vi "PH_gentec_M-Link.Action get Info.vi"(0 "i ref in":refnum<vi>, 5 "error in":errorcluster) -> (14 "i ref out":refnum<vi>, 19 "error out":errorcluster)   [LabVIEW 2014, in "PH_gentec_M-Link.lvlib"]
doc: "This VI gets the basic information from the device."
uses:
  PH_gentec_M-Link.lvlib
  non_GPL/instr.lib/gentec-M-LINK/Driver/Type Defs/gentec-M-Link.Sensor Type.ctl
  non_GPL/instr.lib/gentec-M-LINK/Driver/Type Defs/gentec-M-Link.Range.ctl
  non_GPL/instr.lib/gentec-M-LINK/Driver/Type Defs/gentec-M-Link.Queries with String Answers.ctl
  non_GPL/instr.lib/gentec-M-LINK/Driver/Type Defs/gentec-M-Link.Range Queries.ctl
  PH_Powermeter_BaseClass/PH_Powermeter_BaseClass.State.ctl
  PH_Powermeter_BaseClass/PH_Powermeter_BaseClass.Head Attributes.ctl
  non_GPL/instr.lib/gentec-M-LINK/gentec-M-Link - Driver.lvlib
  PH_Powermeter_BaseClass/PH_Powermeter_BaseClass.lvlib
panel:
  in  "Dummy":T1 items=["1f", "3f", "10f", "30f", "100f", "300f", "1p", "3p", "10p", "30p", "100p", "300p", "1n", "3n", "10n", "30n", "100n", "300n", "1u", "3u", "10u", "30u", "100u", "300u", "1m", "3m", "10m", "30m", "100m", "300m", "1", "3", "10", "30", "100", "300", "1K", "3K", "10K", "30K", "100K", "300K", "1M", "3M", "10M", "30M", "100M", "300M"]
  in  "Sensor Type":T2=1 items=["unknown", "Radiometer", "Joule Meter", "Optical Power", "Thermopyle Power"]
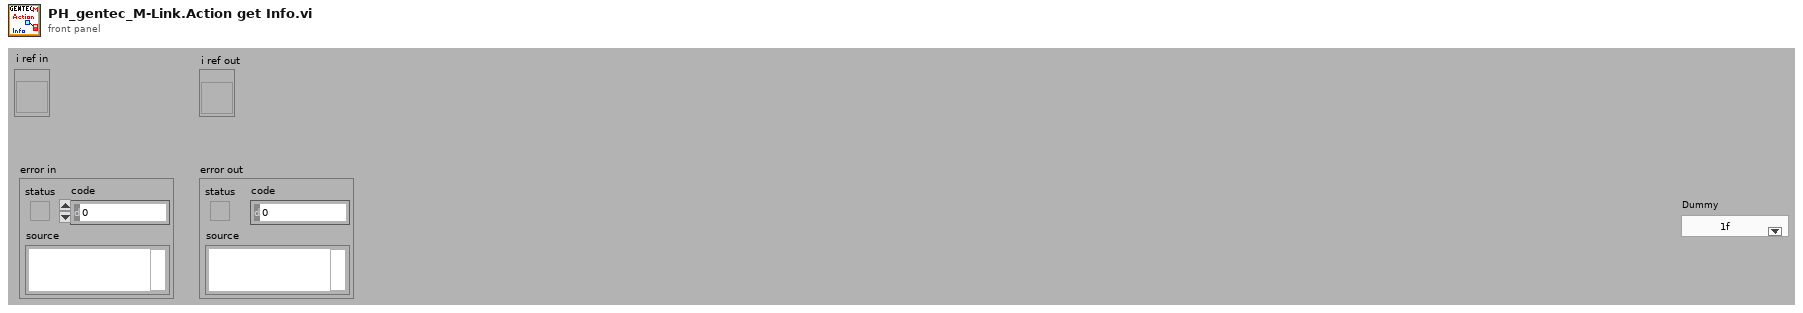
[diagram p1: front panel]
types:
  T1 = typedef "gentec-M-Link - Driver.lvlib/gentec-M-Link.Range.ctl" = u16
  T2 = typedef "gentec-M-Link - Driver.lvlib/gentec-M-Link.Sensor Type.ctl" = u16
  T3 = typedef "PH_Powermeter_BaseClass.lvlib/PH_Powermeter_BaseClass.Head Attributes.ctl" = cluster{"Instrument Type":string, "Head Version":string, "Head Name":string, "Serial Number":string, "Firmware":string, "Sensor Type":string, "MinimumRange":u32, "Maximum Range":u32, "Min Wavelength":i32, "Max Wavelength":i32}
  T4 = typedef "PH_Powermeter_BaseClass.lvlib/PH_Powermeter_BaseClass.State.ctl" = enum32{"off", "operating", "opened", "checked", "connected", "Sets to change", "running"}
  T5 = typedef "gentec-M-Link - Driver.lvlib/gentec-M-Link.Range Queries.ctl" = string
  T6 = typedef "gentec-M-Link - Driver.lvlib/gentec-M-Link.Queries with String Answers.ctl" = string
  T7 = typedef "PH_Powermeter_BaseClass.lvlib/PH_Powermeter_BaseClass.i attribute.ctl" = cluster{"GUI References":T8, "Connection":T9, "Head Attributes":T3, "VISA resource":refnum<visa-resource-name>, "Energy":T10, "Service ID Energy":i32, "Wanted Settings":T11, "Current Settings":T11}
  T8 = typedef "PH_Powermeter_BaseClass.lvlib/PH_Powermeter_BaseClass.GUI Refs.ctl" = cluster{"Head Attributes":refnum<vi>, "Energy":refnum<vi>, "Connection":refnum<vi>, "VISA Resource":refnum<vi>, "Energy evolution":refnum<vi>, "Scaling Factor":refnum<vi>, "Range":refnum<vi>, "Wavelength":refnum<vi>, "Trigger Level":refnum<vi>, "Wanted Settings":refnum<vi>, "Current Settings":refnum<vi>}
  T9 = typedef "PH_Powermeter_BaseClass.lvlib/PH_Powermeter_BaseClass.Connection.ctl" = cluster{"failed checks":i8, "Timeout":bool, "Data read":string, "Failure":bool, "Error":bool, "State":T4}
  T10 = typedef "PH_Powermeter_BaseClass.lvlib/PH_Powermeter_BaseClass.Energy.ctl" = cluster{"current Value":dbl, "unscaled":dbl, "Scaling Factor":dbl}
  T11 = typedef "PH_Powermeter_BaseClass.lvlib/PH_gentec_BaseClass.Head Settings.ctl" = cluster{"Trigger Level":dbl, "Wavelength":u32, "Range":u32}
  T12 = typedef "LVStringsAndValuesArrayTypeDef_U16.ctl" = cluster{"String":string, "Value":u16}[]
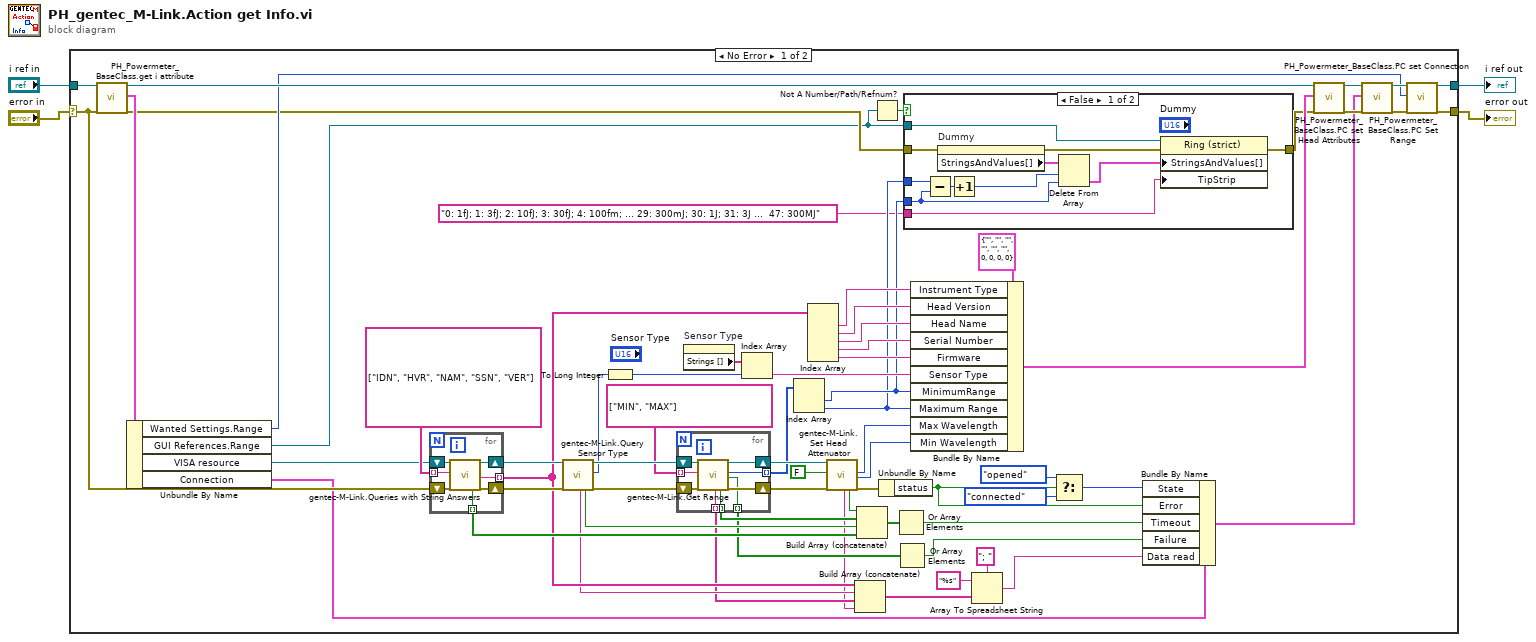
[diagram p0: block diagram]
diagram:
  n1 = case shown="No Error" "error in" {
    selector: "error in" -> [w26 w99]
    tunnel: [w15 w99] -> w3
    tunnel: "i ref in" -> [w27 w98]
    tunnel: [w13 w98] -> w1
    frame No Error {
      n2 = call "PH_Powermeter_BaseClass.get i attribute.vi"("i ref in"=w27, "error in (no error)"=w26) -> ("i ref out"=w25:refnum<vi>, "i attribute"=w20:T7, "error out"=w11:errorcluster)  [unwired: 15 in]
      n3 = Unbundle By Name(w20) -> ("Wanted Settings.Range"=w12:u32, "GUI References.Range"=w6:refnum<vi>, "VISA resource"=w19:refnum<visa-resource-name>, "Connection"=w18:T9)
      n4 = for {
        shift-right: [w97] -> w69
        shift-left: w26 -> [w96]
        shift-right: [w94] -> w68
        shift-left: w19 -> [w95]
        tunnel: [w93] -> w61 mode=indexing
        tunnel: T6[] ["IDN", "HVR", "NAM", "SSN", "VER"] -> [w92] mode=indexing
        tunnel: [w91] -> w43 mode=indexing
        n5 = call "gentec-M-Link.Queries with String Answers.vi"("VISA resource In"=w95, "Queries with String Answers"=w92, "error in (no error)"=w96) -> ("Read Timeout"=w93:bool, "VISA resource Out"=w94:refnum<visa-resource-name>, "Answer"=w91:string, "error out"=w97:errorcluster)  [unwired: 13 in]
      }
      n6 = call "gentec-M-Link.Query Sensor Type.vi"("VISA resource In"=w68, "error in (no error)"=w69) -> ("Data Read"=w42:string, "Read Timeout"=w60:bool, "VISA resource Out"=w67:refnum<visa-resource-name>, "Sensor Type"=w34:T2, "error out"=w65:errorcluster)  [unwired: 13 in]
      n7 = To Long Integer(number=w34) -> (32bit integer=w32:i32)
      n8 = for {
        shift-right: [w89] -> w66
        shift-left: w67 -> [w90]
        shift-right: [w87] -> w64
        shift-left: w65 -> [w88]
        tunnel: [w86] -> w59 mode=indexing
        tunnel: T5[] ["MIN", "MAX"] -> [w85] mode=indexing
        tunnel: [w84] -> w46 mode=indexing
        tunnel: [w83] -> w45 mode=indexing
        tunnel: [w82] -> w41 mode=indexing
        n9 = call "gentec-M-Link.Get Range.vi"("VISA resource In"=w90, "Range Queries"=w85, "error in (no error)"=w88) -> ("Data Read"=w82:string, "Read Timeout"=w86:bool, "VISA resource Out"=w89:refnum<visa-resource-name>, "Range"=w84:T1, "Error"=w83:bool, "error out"=w87:errorcluster)  [unwired: 11 in]
      }
      n10 = property on="Sensor Type" class="Ring (strict)"() -> ("Strings []"=w35:string[])  [unwired: 2 in, 2 out]
      n11 = Index Array(array=w35, index=w32) -> (element=w33:string)
      n12 = Index Array(array=w46) -> (element #1=w9:T1, element #2=w8:T1)  [unwired: 2 in]
      n13 = Index Array(array=w43) -> (element #1=w53:string, element #2=w52:string, element #3=w51:string, element #4=w50:string, element #5=w49:string)  [unwired: 5 in]
      n14 = call "gentec-M-Link.Set Head Attenuator.vi"("VISA resource In"=w66, "Set Head Attenuator"=FALSE, "error in (no error)"=w64) -> ("Data Read"=w40:string, "Read Timeout"=w58:bool, "Max Lambda"=w47:i32, "Min Lambda"=w48:i32, "error out"=w62:errorcluster)  [unwired: 11 in, 1 out]
      n15 = Build Array (concatenate)(w43, w42, w41, w40) -> (w39:string[])
      n16 = Build Array (concatenate)(w58, w59, w60, w61) -> (w57:bool[])
      n17 = Not A Number/Path/Refnum?(number/path/refnum=w6) -> (NaN/Path/Refnum?=w7:bool)
      n18 = Unbundle By Name(w62) -> ("status"=w31:bool)
      n19 = Or Array Elements(Boolean array=w57) -> (logical OR=w56:bool)
      n20 = Or Array Elements(Boolean array=w45) -> (logical OR=w44:bool)
      n21 = case shown="False" w7 {
        tunnel: [w80 w81] -> w10
        tunnel: w6 -> [w79 _]
        tunnel: w11 -> [w78 w81]
        tunnel: w9 -> [w72 _]
        tunnel: w8 -> [w75 _]
        tunnel: "0: 1fJ; 1: 3fJ; 2: 10fJ; 3: 30fJ; 4: 100fm; ... 29: 300mJ; 30: 1J; 31: 3J ...  47: 300MJ" -> [w70 _]
        frame False {
          n22 = Subtract(x=w75, y=w72) -> (x-y=w74:T1)
          n23 = property on="Dummy" class="Ring (strict)"(error in=w78) -> (error out=w77:errorcluster, "StringsAndValues[]"=w76:T12)  [unwired: 1 in, 1 out]
          n24 = Increment(x=w74) -> (x+1=w73:T1)
          n25 = Delete From Array(array=w76, length=w73, index=w72) -> (deleted portion=w71:T12)  [unwired: 1 out]
          n26 = property class="Ring (strict)"(reference=w79, error in=w77, "StringsAndValues[]"=w71, "TipStrip"=w70) -> (error out=w80:errorcluster)  [unwired: 1 out]
        }
        frame True {
        }
      }
      n27 = Bundle By Name(cluster=T3 {"Instrument Type"="", "Head Version"="", "Head Name"="", "Serial Number"="", "Firmware"="", "Sensor Type"="", "MinimumRange"=0, "Maximum Range"=0, "Min Wavelength"=0, "Max Wavelength"=0} ("Head Attributes"), "Instrument Type"=w53, "Head Version"=w52, "Head Name"=w51, "Serial Number"=w50, "Firmware"=w49, "Sensor Type"=w33, "MinimumRange"=w9, "Maximum Range"=w8, "Max Wavelength"=w47, "Min Wavelength"=w48) -> (w16:T3)
      n28 = Array To Spreadsheet String(delimiter (Tab)="; ", array=w39, 3:"%s" ("format string")) -> (spreadsheet string=w36:string)
      n29 = Select(t=PH_Powermeter_BaseClass.State."opened" ("State"), s=w31, f=PH_Powermeter_BaseClass.State."connected") -> (s? t:f=w29:T4)
      n30 = Bundle By Name(cluster=w18, "State"=w29, "Error"=w31, "Timeout"=w56, "Failure"=w44, "Data read"=w36) -> (w21:T9)
      n31 = call "PH_Powermeter_BaseClass.PC set Head Attributes.vi"("VI in"=w25, "Head Attributes"=w16, "error in (no error)"=w10) -> ("VI out"=w24:refnum<vi>, "error out"=w23:errorcluster)  [unwired: 15 in]
      n32 = call "PH_Powermeter_BaseClass.PC set Connection.vi"("VI in"=w24, "Connection"=w21, "error in (no error)"=w23) -> ("VI out"=w14:refnum<vi>, "error out"=w22:errorcluster)  [unwired: 15 in]
      n33 = call "PH_Powermeter_BaseClass.PC Set Range.vi"("VI in"=w14, "Wanted Range"=w12, "error in (no error)"=w22) -> ("VI out"=w13:refnum<vi>, "error out"=w15:errorcluster)  [unwired: 15 in]
    }
    frame Error {
    }
  }
  "error out" <- w3
  "i ref out" <- w1
